vi "Create Group.vi"(8 "error in (no error)":errorcluster, 10 "Group name":string, 11 "Location id in":i32) -> (0 "error out":errorcluster, 3 "Group id":i32)   [LabVIEW 2010, in "HDF5Tools.lvlib"]
uses:
  HDF5Tools.lvlib
  Release/HDF5Tools.dll
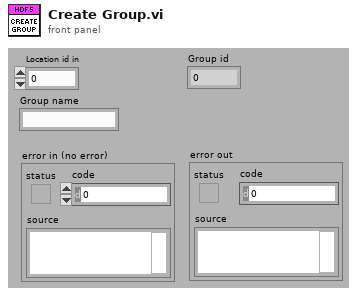
[diagram p1: front panel]
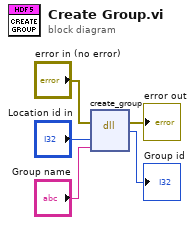
[diagram p0: block diagram]
diagram:
  n1 = dll-call lib="Z:/libraries/HDF5Tools/Release/HDF5Tools.dll" fn="create_group"(error in="error in (no error)", "loc_id"="Location id in", "name"="Group name") -> (error out=→"error out":errorcluster, "group_id"=→"Group id":i32)  [unwired: 4 in, 1 out]
